vi "SetTimeout.vi"(8 "error in (no error)":errorcluster, 10 "Numeric":dbl, 11 "PCO in":refnum<class "PCO_Camera.lvclass">) -> (0 "error out":errorcluster, 3 "PCO out":refnum<class "PCO_Camera.lvclass">)   [LabVIEW 2020, in "PCO_Camera.lvclass"]
uses:
  PCO_Camera.lvclass
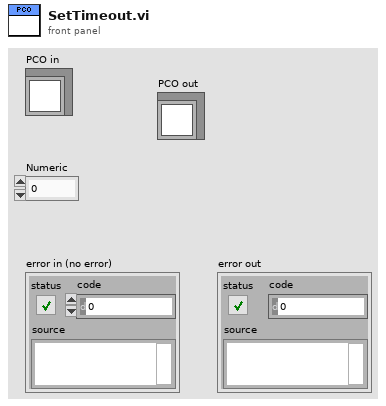
[diagram p1: front panel]
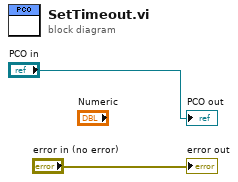
[diagram p0: block diagram]
diagram:
  "error out" <- "error in (no error)"
  "PCO out" <- "PCO in"
